vi "PT1.vi"(0 "input u(k)":dbl, 2 "initialize":bool, 5 "G":dbl, 7 "T1":dbl, 11 "error in (no error)":errorcluster) -> (6 "output y(k)":dbl, 15 "error out":errorcluster)   [LabVIEW 2022 SP3, in "AnalogSignalProcessClass.lvclass"]
uses:
  AnalogSignalProcessClass.lvclass
  <vilib>/addons/Control Design/_Model Construction/Model Typedefs.llb/CD Transfer Function Model (SISO).ctl
  <vilib>/addons/Control Design/_Model Construction/Data Typedefs.llb/CD CtoD Conversion Method.ctl
  <vilib>/addons/Control Design/_Utility/Rendering.llb/Rendering Transfer Function Options.ctl
  <vilib>/Simulation/DiscreteLinear/Implementation/NILVSim Discrete Transfer Function Direct.llb/SIM Discrete Transfer Function Diagram (SISO CD).vi
  <vilib>/Simulation/ContinuousLinear/Implementation/Shared/SIM Transfer Function Support.llb/SIM Convert CD TF to SIM (SISO).vi
  <vilib>/Simulation/ContinuousLinear/Implementation/Shared/SIM Transfer Function Support.llb/SIM TransferFunction Normalize to Buffer.vi
  <vilib>/Simulation/DiscreteLinear/Implementation/Shared/SIM Init Discrete States.vi
  <vilib>/Simulation/DiscreteLinear/Implementation/NILVSim Discrete Transfer Function Direct.llb/SIM Transfer Function Direct core (SISO).vi
  <vilib>/Simulation/ContinuousLinear/Implementation/Shared/SIM Transfer Function Support.llb/SIM TransferFunction Normalize.vi
  <vilib>/Simulation/Implementation/Shared/SIM Polynomials.llb/SIM Remove Zero Coefficients (DBL).vi
  <vilib>/addons/Control Design/_Model Construction/Model Creation.llb/Model Creation SubVI/cd_Create Transfer Function Model.vi
  <vilib>/addons/Control Design/_Frequency Response Analysis/Frequency Response.llb/Frequency Response subVI/cd_Bode (Transfer Function).vi
  <vilib>/addons/Control Design/_Time Response Analysis/Time Response.llb/Time Response subVI/cd_Step Response (Transfer Function).vi
  <vilib>/addons/Control Design/_Model Conversions/Continuous and Discrete.llb/Continuous and Discrete SubVI/cd_Convert Continuous to Discrete (TF).vi
  <vilib>/addons/Control Design/_Utility/Model Viewer.llb/Model Viewer SubVI/cd_Draw Transfer Function Equation (TF).vi
  <vilib>/Simulation/Implementation/Shared/SIM Polynomials.llb/SIM Divide Polynomials (DBL).vi
  <vilib>/Simulation/Implementation/Shared/SIM BuildSimErr.vi
  <vilib>/Simulation/Implementation/XNodeFramework/SimXNode/SimX.xnode
  <vilib>/addons/Control Design/_Model Construction/Model Typedefs.llb/CD Transfer Function Model (MIMO).ctl
  <vilib>/addons/Control Design/_Model Construction/Model Typedefs.llb/CD General Elements.ctl
  <vilib>/addons/Control Design/_Model Conversions/NI_CD_Continuous and Discrete.lvlib
  <vilib>/addons/Control Design/_Model Construction/NI_LinSys_Data Typedefs.lvlib
  <vilib>/addons/Control Design/_Model Construction/NI_LinSys_Model Creation.lvlib
  <vilib>/addons/Control Design/_Utility/NI_CD_Model Viewer.lvlib
  <vilib>/addons/Control Design/_Utility/NI_LinSys_Rendering.lvlib
  <vilib>/addons/Control Design/_Model Construction/NI_LinSys_Model Typedefs.lvlib
  <vilib>/addons/Control Design/_Frequency Response Analysis/NI_CD_Frequency Response.lvlib
  <vilib>/addons/Control Design/_Time Response Analysis/NI_CD_Time Response.lvlib
panel:
  out "Step Response Graph":cluster{"time":dbl[], dbl[]}[](graph)
  out "S Transf":picture
  out "Phase":cluster{"W":dbl[], "Magnitude":dbl[]}(graph)
  out "Magnitude":cluster{"W":dbl[], "Magnitude":dbl[]}(graph)
  out "element":T1 {"delay" format="%.4f"; "Denominator" format="%#_3g"; "Numerator" format="%#_3g"}
  out "Z Transf":picture
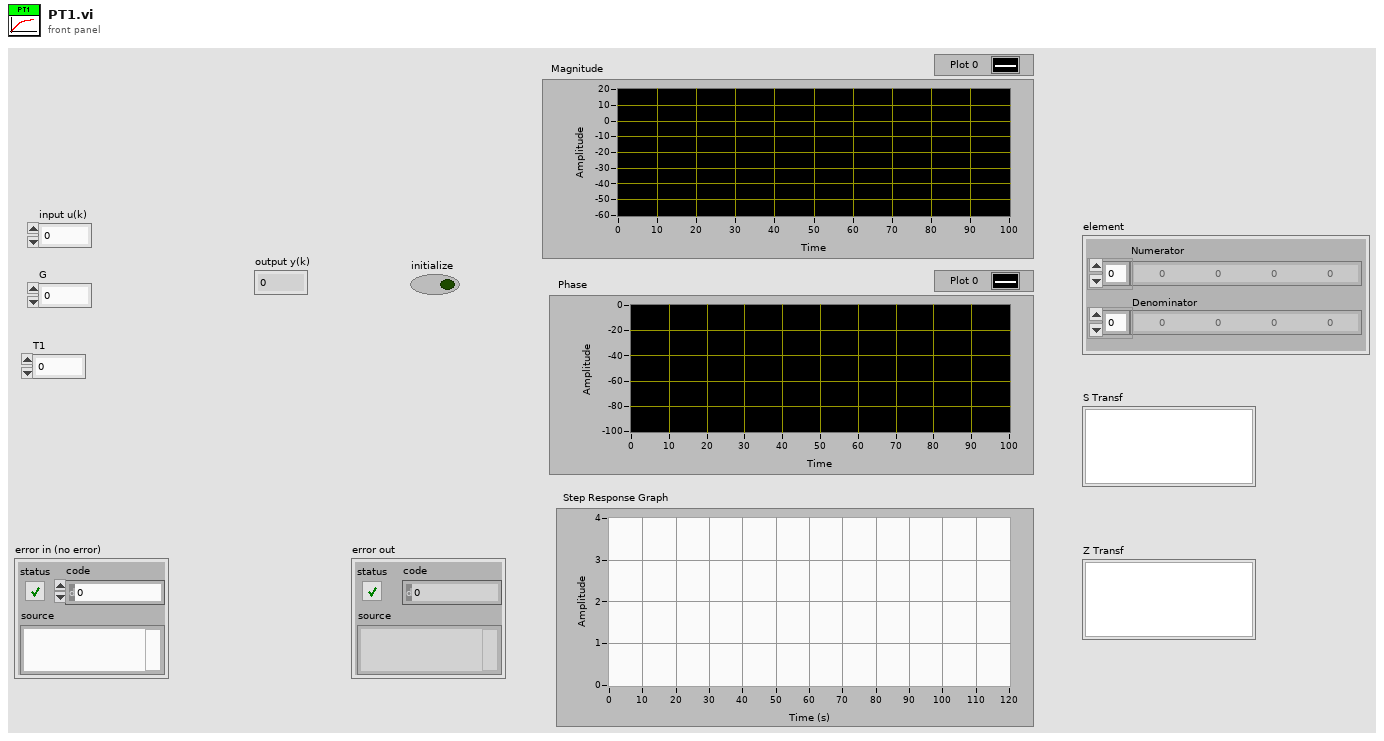
[diagram p1: front panel]
types:
  T1 = typedef "NI_LinSys_Model Typedefs.lvlib/CD Transfer Function Model (SISO).ctl" = cluster{"Numerator":dbl[], "Denominator":dbl[], "delay":dbl}
  T2 = typedef "NI_LinSys_Rendering.lvlib/Rendering Transfer Function Options.ctl" = u16
  T3 = typedef "NI_LinSys_Data Typedefs.lvlib/CD CtoD Conversion Method.ctl" = u16
  T4 = typedef "NI_LinSys_Model Typedefs.lvlib/CD Transfer Function Model (MIMO).ctl" = cluster{"properties":T5, "transfer function(s)":T1[][]}
  T5 = typedef "NI_LinSys_Model Typedefs.lvlib/CD General Elements.ctl" = cluster{"Model name":string, "Input names":string[], "Output names":string[], "Input Delays":dbl[], "Output Delays":dbl[], "Sampling Time":dbl, "Notes":string}
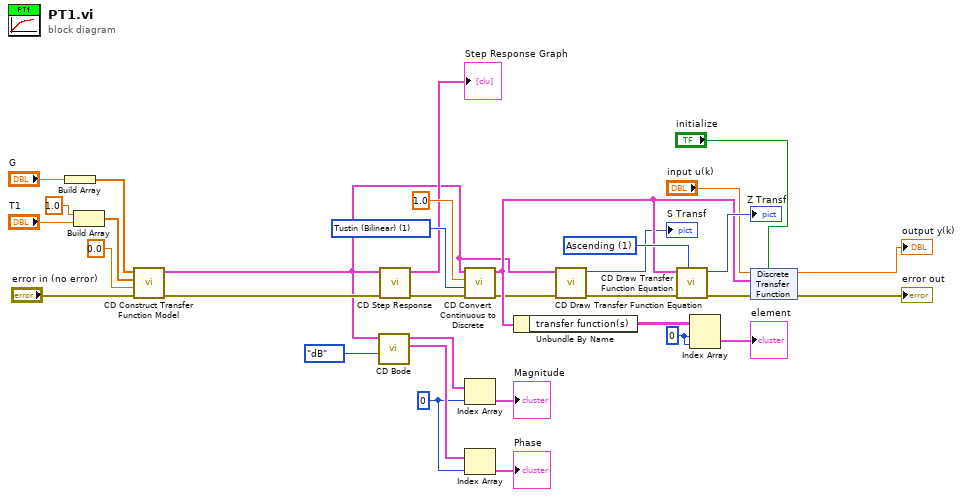
[diagram p0: block diagram]
diagram:
  w18 = 0 ("index")
  w23 = 0 ("index (row)")
  w27 = T2 1 items=["Descending", "Ascending", "Negative Power"] ("Display Format")
  w29 = T3 1 items=["Zero-Order-Hold", "Tustin (Bilinear)", "Prewarp", "Forward", "Backward", "Z-Transform", "First-Order-Hold", "Matched Pole-Zero"] ("Method")
  n1 = Build Array("G") -> (w30:dbl[])
  n2 = Build Array(1.0 ("element"), "T1") -> (w31:dbl[])
  n3 = call-poly <vilib>:"CD Construct Transfer Function Model.vi"("error in (no error)"="error in (no error)", "Delay"=0.0 ("delay"), "Denominator"=w31, "Numerator"=w30) -> ("error out"=w4:errorcluster, "Transfer Function Model"=w1:T4)  [unwired: 6 in]
  n4 = call-poly <vilib>:"CD Bode.vi"("Magnitude Scale"=enum16{"linear", "dB"}."dB", "Transfer Function Model"=w1) -> ("Bode Phase"=w19:cluster{"W":dbl[], "Magnitude":dbl[]}[], "Bode Magnitude"=w20:cluster{"W":dbl[], "Magnitude":dbl[]}[])  [unwired: 5 in, 3 out]
  n5 = call-poly <vilib>:"CD Step Response.vi"("error in (no error)"=w4, "Transfer Function Model"=w1) -> ("error out"=w3:errorcluster, "Step Response Graph"=→"Step Response Graph":cluster{"time":dbl[], dbl[]}[])  [unwired: 7 in, 1 out]
  n6 = call-poly <vilib>:"CD Convert Continuous to Discrete.vi"("error in (no error)"=w3, "Method"=w29, "Sampling Time (s)"=1.0, "Continuous Transfer Function Model"=w1) -> ("error out"=w8:errorcluster, "Discrete Transfer Function Model"=w14:T4)  [unwired: 6 in]
  n7 = Index Array(array=w20, index=w18) -> (element=→"Magnitude":cluster{"W":dbl[], "Magnitude":dbl[]})
  n8 = Index Array(array=w19, index=w18) -> (element=→"Phase":cluster{"W":dbl[], "Magnitude":dbl[]})
  n9 = Unbundle By Name(w14) -> ("transfer function(s)"=w24:T1[][])
  n10 = call-poly <vilib>:"CD Draw Transfer Function Equation.vi"("error in (no error)"=w8, "Transfer Function Model"=w1) -> ("error out"=w7:errorcluster, "Equation"=→"S Transf":picture)  [unwired: 7 in, 1 out]
  n11 = call-poly <vilib>:"CD Draw Transfer Function Equation.vi"("Display Format"=w27, "error in (no error)"=w7, "Transfer Function Model"=w14) -> ("error out"=w11:errorcluster, "Equation"=→"Z Transf":picture)  [unwired: 6 in, 1 out]
  n12 = Index Array(array=w24, index (row)=w23, index (col)=w23) -> (element=→"element":T1)
  n13 = xnode "Discrete Transfer Function"("input u(k)"="input u(k)", "Transfer Function"=w14, "initialize"="initialize", "error in (no error)"=w11) -> ("output y(k)"=→"output y(k)":dbl, "error out"=→"error out":errorcluster)
